vi "Dependency Test VI Template.vi"(8 "Error In":errorcluster) -> (0 "Error Out":errorcluster, 2 "Pass?":bool)   [LabVIEW 2020, in "LMH-Toolbox.lvlib" / "LMH-Installer Tools.lvlib"]
uses:
  LMH-Installer Tools.lvlib
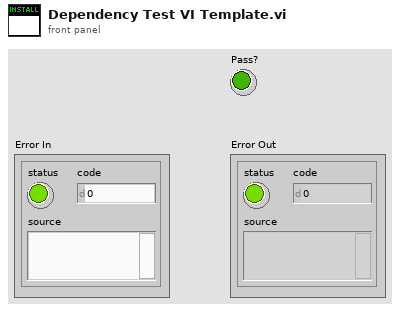
[diagram p1: front panel]
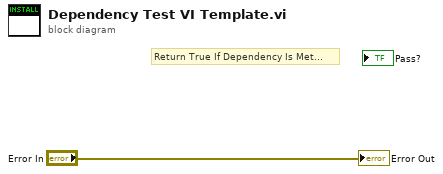
[diagram p0: block diagram]
diagram:
  # "Return True If Dependency Is Met..."
  "Error Out" <- "Error In"
